vi "Get Splash Screen State.vi"(8 "Error In":errorcluster) -> (0 "Error Out":errorcluster, 3 "Close Splash Screen Out":bool)   [LabVIEW 2014]
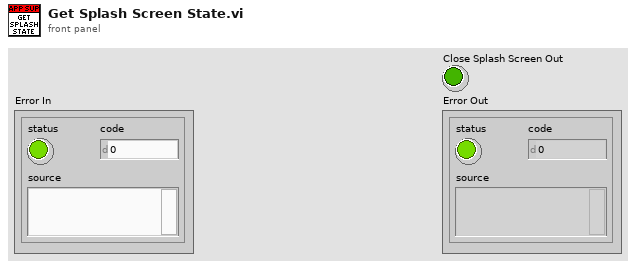
[diagram p1: front panel]
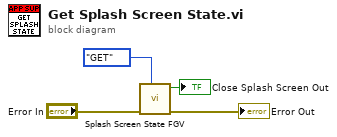
[diagram p0: block diagram]
diagram:
  n1 = call "Splash Screen State FGV.vi"("Operation"=enum16{"GET", "SET"}."GET", "Error In"="Error In") -> ("Error Out"=→"Error Out":errorcluster, "Close Splash Screen Out"=→"Close Splash Screen Out":bool)  [unwired: 8 in]
